vi "ExecutePlay.vi"(0 "object in":refnum<class "PassPlay_v2.lvclass">, 2 "Robots in":refnum<class "Robot.lvclass">[](array[class]), 3 "GameRef":refnum<data-value>, 5 "error in (no error)":errorcluster) -> (14 "object out":refnum<class "PassPlay_v2.lvclass">, 16 "Robots out":refnum<class "Robot.lvclass">[](array[class]), 19 "error out":errorcluster)   [LabVIEW 2023, in "PassPlay_v2.lvclass"]
uses:
  PassPlay_v2.lvclass
  Play_v2_class/Play_v2.lvclass
  Robot_class/Robot.lvclass
  Game_class/Game.lvclass
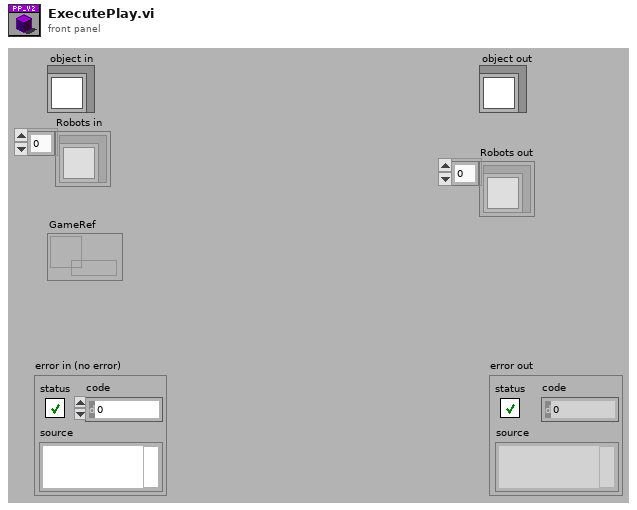
[diagram p1: front panel]
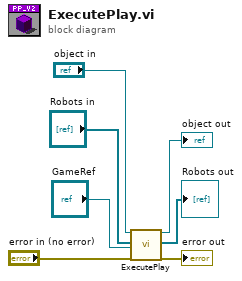
[diagram p0: block diagram]
diagram:
  n1 = call-parent "ExecutePlay.vi"("object in"="object in", "Robots in"="Robots in", "GameRef"="GameRef", "error in (no error)"="error in (no error)") -> ("object out"=→"object out":refnum<class "PassPlay_v2.lvclass">, "Robots out"=→"Robots out":refnum<class "Robot.lvclass">[], "error out"=→"error out":errorcluster)  [unwired: 13 in]
